vi "GetActualValues.vi"(5 "error in (no error)":errorcluster) -> (16 "ActualValues":cluster{"T":dbl, "RH":dbl} {"RH" format="%.2f"; "T" format="%.2f"}, 19 "error out":errorcluster)   [LabVIEW 2019, in "WebServiceData.lvclass"]
uses:
  WebServiceData.lvclass
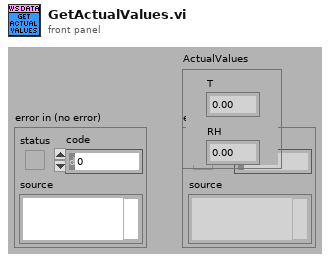
[diagram p1: front panel]
types:
  T1 = typedef "WebServiceData.lvclass/ObjectAttributes.ctl" = cluster{"ActualValues":cluster{"T":dbl, "RH":dbl}}
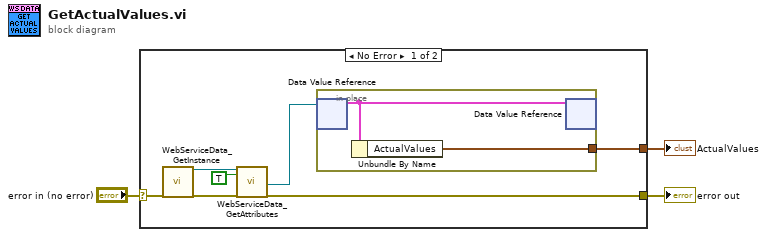
[diagram p0: block diagram]
diagram:
  n1 = case shown="No Error" "error in (no error)" {
    selector: "error in (no error)" -> [w8 w13]
    tunnel: [w10 w13] -> w2
    tunnel: [w4 _] -> w1
    frame No Error {
      n2 = call "WebServiceData_GetInstance.vi"("error in (no error)"=w8) -> ("reference out"=w9:refnum<class "WebServiceData.lvclass">, "error out"=w7:errorcluster)  [unwired: 14 in, 3 out]
      n3 = call "WebServiceData_GetAttributes.vi"("reference in"=w9, "OnlyGetDvrReference(False)"=TRUE, "error in (no error)"=w7) -> ("DataRef"=w6:refnum<data-value>, "error out"=w10:errorcluster)  [unwired: 13 in, 2 out]
      n4 = in-place {
        in-place-border: [w12] -> w4
        n5 = in-place-dvr #1(w6) -> (w11:T1)  [unwired: 1 out]
        n6 = Unbundle By Name(w11) -> ("ActualValues"=w12:cluster{"T":dbl, "RH":dbl})
        n7 = in-place-dvr #1(w11) -> ()  [unwired: 2 out]
      }
    }
    frame Error {
    }
  }
  "error out" <- w2
  "ActualValues" <- w1
